vi "extractSSIEncoderData.vi"(8 "error in (no error)":errorcluster, 11 "ILC in":refnum<class "ILC.lvclass">) -> (0 "error out":errorcluster, 3 "ILC out":refnum<class "ILC.lvclass">)   [LabVIEW 2015, in "ILCCommon.lvlib" / "ILC.lvclass"]
uses:
  <userlib>/Common/ILC/ILC/ILC.lvclass
  <userlib>/Common/ILC/ILCModelTypedefs/FinalDelimiter.ctl
  <userlib>/Common/ILC/ILC/ILC.lvclass/ILC.ctl
  <userlib>/Common/ILC/ILCModelTypedefs/ILCModelTypedefs.lvlib
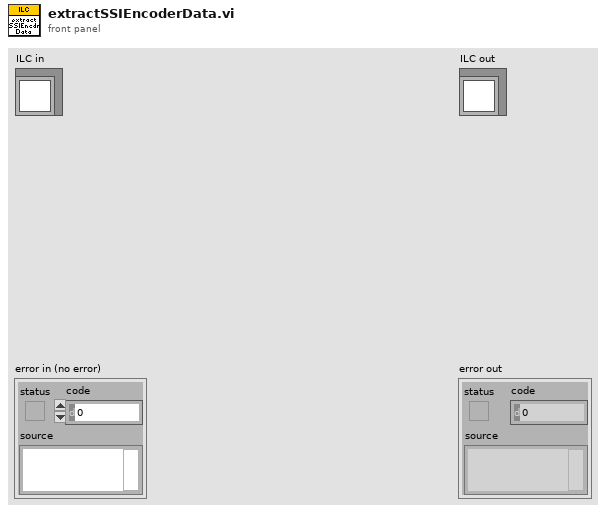
[diagram p1: front panel]
types:
  T1 = typedef "ILCCommon.lvlib/ILCModelTypedefs.lvlib/FinalDelimiter.ctl" = enum16{",", "<CR><LF>"}
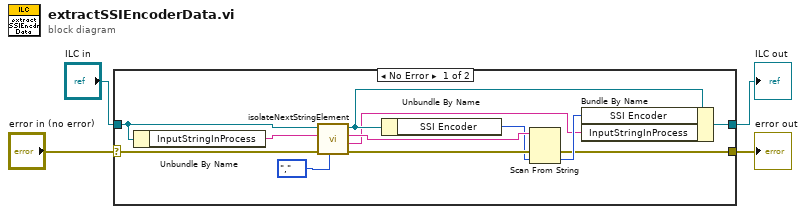
[diagram p0: block diagram]
diagram:
  n1 = case shown="No Error" "error in (no error)" {
    selector: "error in (no error)" -> [w10 w18]
    tunnel: [w9 w18] -> w3
    tunnel: [w11 w17] -> w1
    tunnel: "ILC in" -> [w7 w17]
    frame No Error {
      n2 = Unbundle By Name(w7) -> ("InputStringInProcess"=w8:string)
      n3 = call <userlib>:"isolateNextStringElement.vi"("Final Delimiter"=FinalDelimiter.",", "error in (no error)"=w10, "inputString"=w8, "ILC in"=w7) -> ("error out"=w15:errorcluster, "remainingString"=w5:string, "extractedSegment"=w16:string, "ILC out"=w6:refnum<class "ILC.lvclass">)  [unwired: 4 in]
      n4 = Unbundle By Name(w6) -> ("SSI Encoder"=w12:i32)
      n5 = Scan From String(input string=w16, error in=w15, default 1=w12) -> (error out=w9:errorcluster, output 1=w13:i32)  [unwired: 2 in, 2 out]
      n6 = Bundle By Name(cluster=w6, "SSI Encoder"=w13, "InputStringInProcess"=w5) -> (w11:refnum<class "ILC.lvclass">)
    }
    frame Error {
    }
  }
  "error out" <- w3
  "ILC out" <- w1
